vi "calc_spiral_for_lookup.vi"(6 "error in":errorcluster, 7 "All scan parameters":T1={"Fiber parameters"={"Frequency"=100.0, "Amplitude X"=0.0, "Amplitude Y"=0.0, "Initial Amplitude X"=0.0, "Initial Amplitude Y"=0.0, "Phase"=0.0}, "Spiral parameters"={"Imaging periods"=1.0, "Settling periods"=1.0, "Resting periods"=1.0}, "Run parameters"={"Run mode"=enum."Continuous", "Averages per frame"=1, "No. of frames"=1}, "Acquisition parameters"={"Cycles per pixel"=0, "Image size"=1, "Bidirectional acquisition"=FALSE}, "Fiber parameters pixel_mapper"={"Frequency"=1.0, "Amplitude X"=1.0, "Amplitude Y"=1.0, "Initial Amplitude X"=0.0, "Initial Amplitude Y"=0.0, "Phase"=0.0}, "Smooth_coeffs_cluster"={"Coeff 1"=0.0, "Coeff 2"=0.0}, "Storage parameters"={"Autosave"=FALSE, "Path"=path ""}, "Mapping corrections"={"Phase increase"=0.0, "Amplitude correction"=0.0}} {"Mapping corrections"."Phase increase" min=-1.0 max=1.0 step=0.01; "Smooth_coeffs_cluster"."Coeff 1" min=0.0 max=1.0 step=0.05; "Smooth_coeffs_cluster"."Coeff 2" min=0.0 max=1.0 step=0.05; "Fiber parameters pixel_mapper"."Phase" min=-90.0 max=90.0 step=5.0; "Fiber parameters pixel_mapper"."Initial Amplitude Y" min=0.0 max=1.0 step=0.1; "Fiber parameters pixel_mapper"."Initial Amplitude X" min=0.0 max=1.0 step=0.1; "Fiber parameters pixel_mapper"."Amplitude Y" min=0.0 max=3.0 step=0.1; "Fiber parameters pixel_mapper"."Amplitude X" min=0.0 max=3.0 step=0.1; "Fiber parameters pixel_mapper"."Frequency" min=100.0 max=6000.0 step=1.0; "Acquisition parameters"."Image size" items=["128x128 px"=128, "256x256 px"=256, "512x512 px"=512]; "Acquisition parameters"."Cycles per pixel" min=100 max=90000 step=1; "Run parameters"."No. of frames" min=1 max=1000 step=1; "Run parameters"."Averages per frame" min=1 max=32; "Spiral parameters"."Resting periods" min=10.0 max=1000.0 step=1.0; "Spiral parameters"."Settling periods" min=1.0 max=1000.0 step=1.0; "Spiral parameters"."Imaging periods" min=1.0 max=1000.0 step=1.0; "Fiber parameters"."Phase" min=-90.0 max=90.0 step=5.0; "Fiber parameters"."Initial Amplitude Y" min=0.0 max=1.0 step=0.1; "Fiber parameters"."Initial Amplitude X" min=0.0 max=1.0 step=0.1; "Fiber parameters"."Amplitude Y" min=0.0 max=3.0 step=0.1; "Fiber parameters"."Amplitude X" min=0.0 max=3.0 step=0.1; "Fiber parameters"."Frequency" min=100.0 max=6000.0 step=1.0}, 8 "Lookup array parameter cluster":T11 {"Pixels per spiral" min=1 max=90000 step=1}, 9 "Lookup array memref in":refnum<data-value>) -> (0 "error out":errorcluster, 1 "Phase correction":dbl[](array[numeric]), 2 "Amplitude correction":dbl[](array[numeric]), 3 "Lookup array memref out":refnum<data-value>)   [LabVIEW 2011, in "Fiberscope_library.lvlib"]
uses:
  Fiberscope_library.lvlib
  typedefs/lookup_array_parameter_cluster.ctl
  typedefs/pixel_per_spiral_I32.ctl
  typedefs/all_scan_parameters_cluster.ctl
  typedefs/fiber_parameters_cluster.ctl
  typedefs/spiral_parameters_cluster.ctl
  typedefs/run_parameters_cluster.ctl
  typedefs/run_mode_enum.ctl
  typedefs/acquisition_parameters_cluster.ctl
  typedefs/image_size_I32.ctl
  typedefs/smooth_coeffs_cluster.ctl
  typedefs/storage_parameters_cluster.ctl
  typedefs/mapping_corrections_cluster.ctl
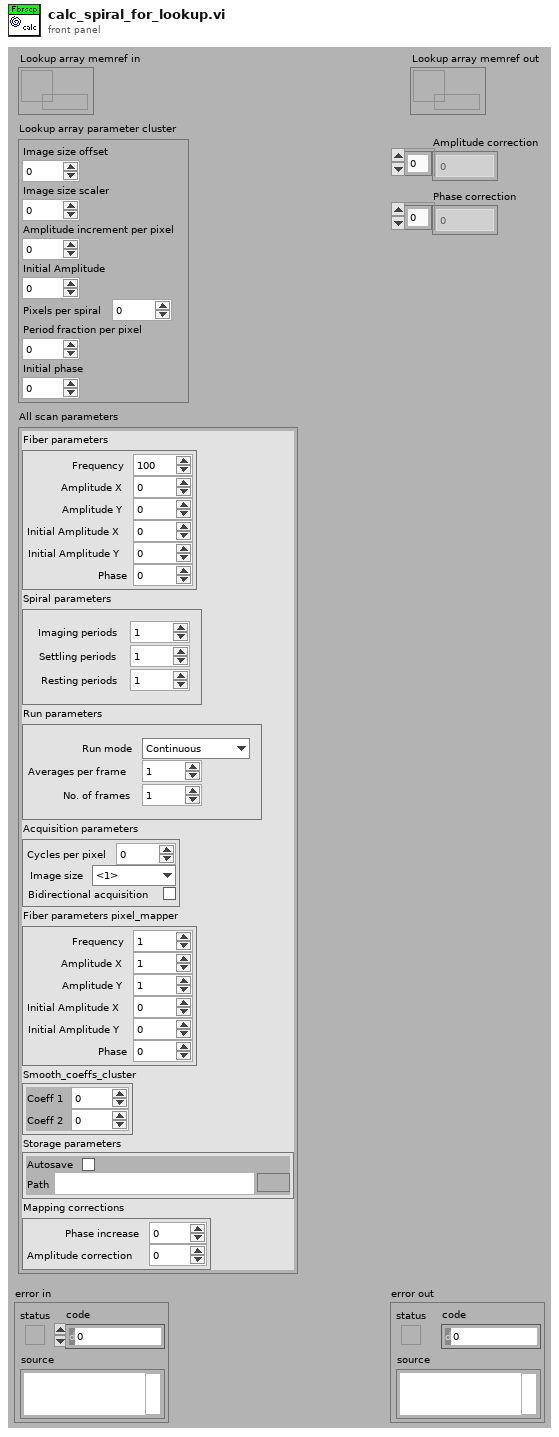
[diagram p1: front panel]
types:
  T1 = typedef "Fiberscope_library.lvlib/all_scan_parameters_cluster.ctl" = cluster{"Fiber parameters":T2, "Spiral parameters":T3, "Run parameters":T4, "Acquisition parameters":T6, "Fiber parameters pixel_mapper":T2, "Smooth_coeffs_cluster":T8, "Storage parameters":T9, "Mapping corrections":T10}
  T2 = typedef "Fiberscope_library.lvlib/fiber_parameters_cluster.ctl" = cluster{"Frequency":dbl, "Amplitude X":dbl, "Amplitude Y":dbl, "Initial Amplitude X":dbl, "Initial Amplitude Y":dbl, "Phase":dbl}
  T3 = typedef "Fiberscope_library.lvlib/spiral_parameters_cluster.ctl" = cluster{"Imaging periods":dbl, "Settling periods":dbl, "Resting periods":dbl}
  T4 = typedef "Fiberscope_library.lvlib/run_parameters_cluster.ctl" = cluster{"Run mode":T5, "Averages per frame":u8, "No. of frames":u32}
  T5 = typedef "Fiberscope_library.lvlib/run_mode_enum.ctl" = enum16{"Continuous", "Single frame", "No. of frames"}
  T6 = typedef "Fiberscope_library.lvlib/acquisition_parameters_cluster.ctl" = cluster{"Cycles per pixel":u32, "Image size":T7, "Bidirectional acquisition":bool}
  T7 = typedef "Fiberscope_library.lvlib/image_size_I32.ctl" = i32
  T8 = typedef "Fiberscope_library.lvlib/smooth_coeffs_cluster.ctl" = cluster{"Coeff 1":dbl, "Coeff 2":dbl}
  T9 = typedef "Fiberscope_library.lvlib/storage_parameters_cluster.ctl" = cluster{"Autosave":bool, "Path":path}
  T10 = typedef "Fiberscope_library.lvlib/mapping_corrections_cluster.ctl" = cluster{"Phase increase":dbl, "Amplitude correction":dbl}
  T11 = typedef "Fiberscope_library.lvlib/lookup_array_parameter_cluster.ctl" = cluster{"Image size offset":dbl, "Image size scaler":dbl, "Amplitude increment per pixel":dbl, "Initial Amplitude":dbl, "Pixels per spiral":T12, "Period fraction per pixel":dbl, "Initial phase":dbl}
  T12 = typedef "Fiberscope_library.lvlib/pixel_per_spiral_I32.ctl" = i32
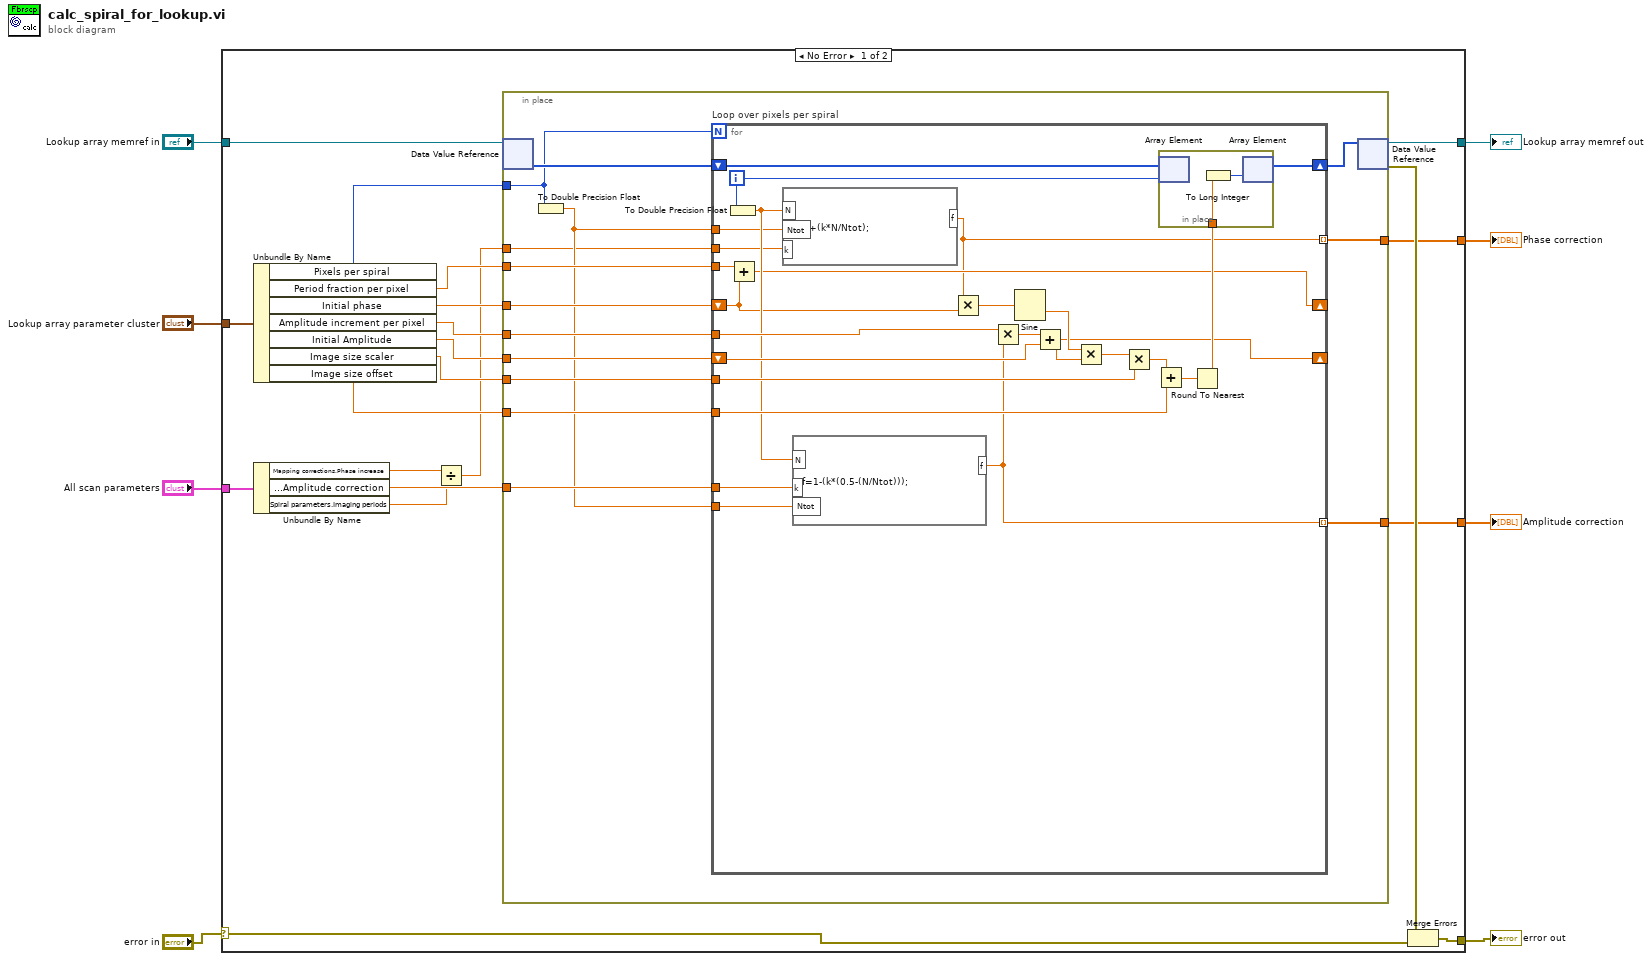
[diagram p0: block diagram]
diagram:
  n1 = case shown="No Error" "error in" {
    selector: "error in" -> [w16 w71]
    tunnel: "Lookup array memref in" -> [w28 w70]
    tunnel: "Lookup array parameter cluster" -> [w27 _]
    tunnel: [w17 w71] -> w5
    tunnel: [w19 w70] -> w4
    tunnel: [w14 _] -> w3
    tunnel: "All scan parameters" -> [w10 _]
    tunnel: [w11 _] -> w1
    frame No Error {
      n2 = Unbundle By Name(w27) -> ("Pixels per spiral"=w26:T12, "Period fraction per pixel"=w25:dbl, "Initial phase"=w24:dbl, "Amplitude increment per pixel"=w23:dbl, "Initial Amplitude"=w22:dbl, "Image size scaler"=w21:dbl, "Image size offset"=w20:dbl)
      n3 = Unbundle By Name(w10) -> ("Mapping corrections.Phase increase"=w13:dbl, "Mapping corrections.Amplitude correction"=w15:dbl, "Spiral parameters.Imaging periods"=w9:dbl)
      n4 = Divide(x=w13, y=w9) -> (x/y=w12:dbl)
      n5 = in-place {
        in-place-border: w25 -> [w32]
        in-place-border: w26 -> [w35]
        in-place-border: w22 -> [w42]
        in-place-border: w23 -> [w41]
        in-place-border: w21 -> [w40]
        in-place-border: w20 -> [w39]
        in-place-border: w24 -> [w37]
        in-place-border: w12 -> [w30]
        in-place-border: w15 -> [w36]
        in-place-border: [w33] -> w14
        in-place-border: [w29] -> w11
        n6 = in-place-dvr #1(w28) -> (w38:i32[])  [unwired: 1 out]
        n7 = To Double Precision Float(number=w35) -> (double precision float=w31:dbl)
        n8 = for "Loop over pixels per spiral" {
          N: w35 -> [_]
          shift-right: [w44] -> _
          shift-left: w37 -> [w46]
          tunnel: w32 -> [w58]
          shift-right: [w52] -> _
          shift-left: w42 -> [w55]
          tunnel: w41 -> [w51]
          tunnel: w40 -> [w65]
          tunnel: w39 -> [w63]
          shift-right: [w59] -> w34
          shift-left: w38 -> [w61]
          tunnel: w36 -> [w57]
          tunnel: w31 -> [w56]
          tunnel: [w54] -> w33 mode=indexing
          tunnel: w31 -> [w48]
          tunnel: w30 -> [w47]
          tunnel: [w43] -> w29 mode=indexing
          i -> [w53]
          n9 = To Double Precision Float(number=w53) -> (double precision float=w49:dbl)
          n10 = Add(x=w58, y=w46) -> (x+y=w44:dbl)
          n11 = formula code="f=1+(k*N/Ntot);"("N"=w49, "Ntot"=w48, "k"=w47) -> ("f"=w43:dbl)
          n12 = formula code="f=1-(k*(0.5-(N/Ntot)));"("N"=w49, "k"=w57, "Ntot"=w56) -> ("f"=w54:dbl)
          n13 = Multiply(x=w43, y=w46) -> (x*y=w45:dbl)
          n14 = Multiply(x=w51, y=w54) -> (x*y=w50:dbl)
          n15 = Sine(x=w45) -> (sin(x)=w67:dbl)
          n16 = Add(x=w50, y=w55) -> (x+y=w52:dbl)
          n17 = Multiply(x=w67, y=w52) -> (x*y=w66:dbl)
          n18 = Multiply(x=w66, y=w65) -> (x*y=w64:dbl)
          n19 = Add(x=w64, y=w63) -> (x+y=w62:dbl)
          n20 = Round To Nearest(number=w62) -> (nearest integer value=w60:dbl)
          n21 = in-place {
            in-place-border: w60 -> [w69]
            n22 = in-place-array #2(w61, w53) -> ()  [unwired: 1 out]
            n23 = To Long Integer(number=w69) -> (32bit integer=w68:i32)
            n24 = in-place-array #2(w68) -> (w59:i32[])  [unwired: 1 out]
          }
        }
        n25 = in-place-dvr #1(w34) -> (w19:refnum<data-value>, w18:errorcluster)
      }
      n26 = Merge Errors(w18, w16) -> (w17:errorcluster)
    }
    frame Error {
    }
  }
  "error out" <- w5
  "Lookup array memref out" <- w4
  "Amplitude correction" <- w3
  "Phase correction" <- w1
